vi "Memory.Pointer.Duplicate.vi"(8 "error in (no error)":errorcluster, 11 "pointer in":refnum<class "Memory.Pointer.lvclass">) -> (0 "error out":errorcluster, 2 "new pointer out":refnum<class "Memory.Pointer.lvclass">, 3 "pointer out":refnum<class "Memory.Pointer.lvclass">)   [LabVIEW 2016, in "Memory Manager.lvlib" / "Memory.Pointer.lvclass"]
uses:
  Memory.Pointer.lvclass
  Memory.Pointer.lvclass/Memory.Pointer.ctl
  Memory.Pointer.Copy All.Unsafe.vi
  Accessors/Set Address.vi
  Accessors/Set Size.vi
  Memory.Pointer.Copy.vi
  Memory.Pointer.Copy.Unsafe.vi
  Accessors/Get Address.vi
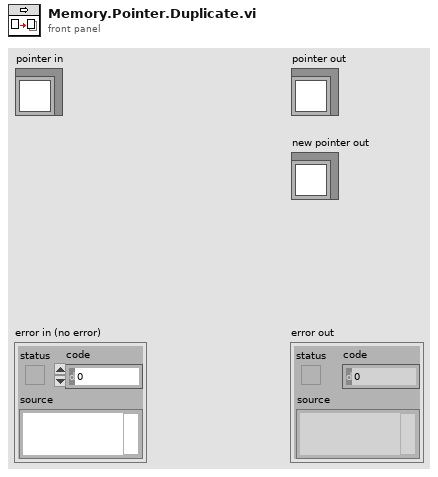
[diagram p1: front panel]
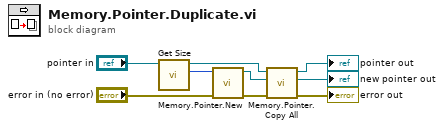
[diagram p0: block diagram]
diagram:
  n1 = call "Get Size.vi"("Pointer in"="pointer in") -> ("size"=w7:u64, "Pointer out"=w4:refnum<class "Memory.Pointer.lvclass">)  [unwired: 8 in, 1 out]
  n2 = call "Memory.Pointer.New.vi"("error in (no error)"="error in (no error)", "size"=w7) -> ("error out"=w6:errorcluster, "pointer"=w5:refnum<class "Memory.Pointer.lvclass">)  [unwired: 8 in]
  n3 = call-poly "Memory.Pointer.Copy All.vi"("error in (no error)"=w6, "dst pointer in"=w5, "src pointer in"=w4) -> ("error out"=→"error out":errorcluster, "dst pointer out"=→"new pointer out":refnum<class "Memory.Pointer.lvclass">, "src pointer out"=→"pointer out":refnum<class "Memory.Pointer.lvclass">)  [unwired: 6 in]
